vi "createSerialCommunicator.vi"(8 "error in (no error)":errorcluster, 10 "Serial Protocol":T1, 11 "SerialCommFactory in":refnum<class "SerialCommFactory.lvclass">) -> (0 "error out":errorcluster, 2 "serialCommunicator":refnum<class "SerialCommunicator.lvclass">, 3 "SerialCommFactory out":refnum<class "SerialCommFactory.lvclass">)   [LabVIEW 2013, in "SerialProtocols.lvlib" / "SerialCommFactory.lvclass"]
uses:
  <userlib>/Common/SerialProtocols/SerialCommFactory/SerialCommFactory/SerialCommFactory.lvclass
  <userlib>/Common/SerialProtocols/SerialCommunicator/SerialCommunicator/SerialCommunicator.lvclass
  <userlib>/Common/SerialProtocols/Configuration/SerialProtocol.ctl
  <userlib>/Common/SerialProtocols/SerialCommunicator/RS232/RS232.lvclass
  <userlib>/Common/SerialProtocols/SerialCommunicator/RS485/RS485.lvclass
  <userlib>/Common/SerialProtocols/SerialCommunicator/SerialSimulator/SerialSimulator.lvclass
  <userlib>/Common/SerialProtocols/SerialProtocols.lvlib
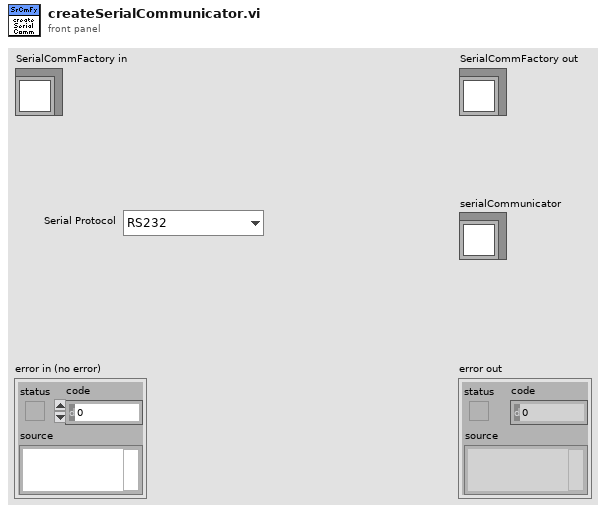
[diagram p1: front panel]
types:
  T1 = typedef "SerialProtocols.lvlib/SerialProtocol.ctl" = enum16{"RS232", "RS485", "SerialSimulator"}
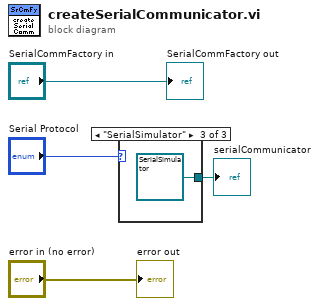
[diagram p0: block diagram]
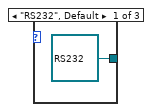
[diagram p2: hidden frame]
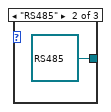
[diagram p3: hidden frame]
diagram:
  n1 = case shown="\"SerialSimulator\"" "Serial Protocol" {
    tunnel: [refnum<class "RS232.lvclass"> refnum ("RS232.lvclass") refnum<class "RS485.lvclass"> refnum ("RS485.lvclass") refnum<class "SerialSimulator.lvclass"> refnum ("SerialSimulator.lvclass")] -> w3
    frame "RS232", Default {
    }
    frame "RS485" {
    }
    frame "SerialSimulator" {
    }
  }
  "serialCommunicator" <- w3
  "error out" <- "error in (no error)"
  "SerialCommFactory out" <- "SerialCommFactory in"
